vi "Calculate Acceleration and PA.vi"(10 "System Weight":dbl, 11 "Force Array":dbl[](array[numeric])) -> (2 "Acceleration Array":dbl[](array[numeric]), 3 "Peak Acceleration":dbl)   [LabVIEW 2016]
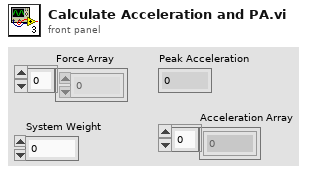
[diagram p1: front panel]
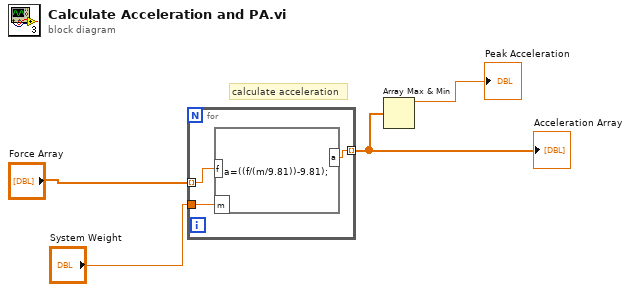
[diagram p0: block diagram]
diagram:
  # "calculate acceleration"
  n1 = for {
    tunnel: "System Weight" -> [w7]
    tunnel: [w6] -> w3 mode=indexing
    tunnel: "Force Array" -> [w5] mode=indexing
    n2 = formula code="a=((f/(m/9.81))-9.81);"("f"=w5, "m"=w7) -> ("a"=w6:dbl)
  }
  "Acceleration Array" <- w3
  n3 = Array Max & Min(array=w3) -> (max value=→"Peak Acceleration":dbl)  [unwired: 3 out]
